vi "ArrayFunctions_CheckForDups(DBL).vi"(1 "Array":dbl[](array[numeric])) -> (15 "DupElements":dbl[](array[numeric]), 16 "DupElements(String)":string, 17 "FoundDups":bool)   [LabVIEW 2016]
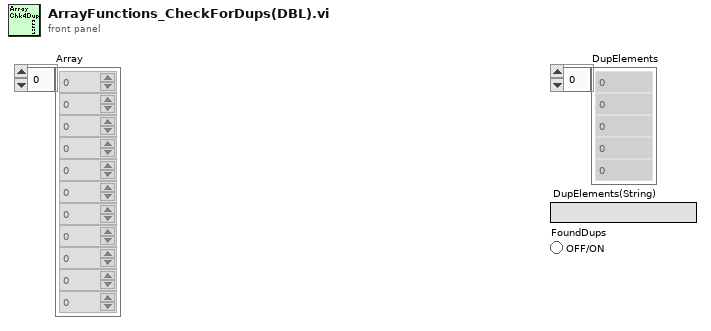
[diagram p1: front panel]
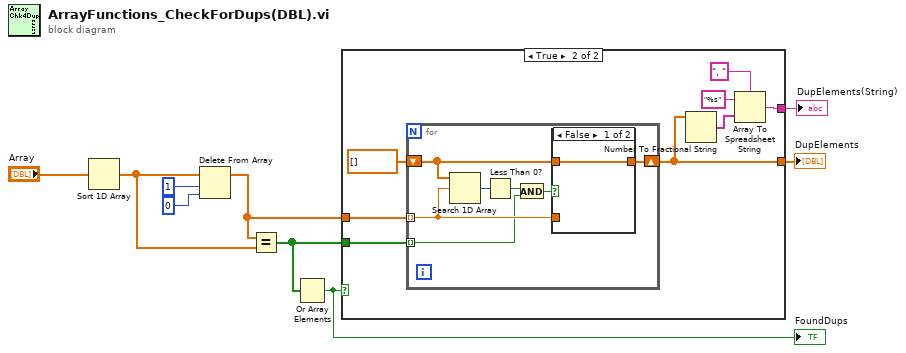
[diagram p0: block diagram]
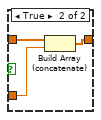
[diagram p3: hidden frame]
diagram:
  n1 = Sort 1D Array(array="Array") -> (sorted array=w2:dbl[])
  n2 = Delete From Array(array=w2, length=1, index=0) -> (array with subset deleted=w7:dbl[])  [unwired: 1 out]
  n3 = Equal?(x=w7, y=w2) -> (x = y?=w6:bool[])
  n4 = Or Array Elements(Boolean array=w6) -> (logical OR=w4:bool)
  "FoundDups" <- w4
  n5 = case shown="True" w4 {
    tunnel: w7 -> [_ w17]
    tunnel: w6 -> [_ w16]
    tunnel: [_ w14] -> w5
    tunnel: [_ w10] -> w1
    frame False {
    }
    frame True {
      n6 = for {
        tunnel: w17 -> [w22] mode=indexing
        tunnel: w16 -> [w18] mode=indexing
        shift-right: [w24] -> w14
        shift-left: dbl[] [] ("array w/ subset deleted") -> [w23]
        n7 = Search 1D Array(1D array=w23, element=w22) -> (index of element=w21:i32)  [unwired: 1 in]
        n8 = Less Than 0?(x=w21) -> (x < 0?=w20:bool)
        n9 = And(x=w20, y=w18) -> (x .and. y?=w19:bool)
        n10 = case shown="False" w19 {
          tunnel: [w25 w28] -> w24
          tunnel: w23 -> [w25 w27]
          tunnel: w22 -> [_ w26]
          frame False {
          }
          frame True {
            n11 = Build Array (concatenate)(w27, w26) -> (w28:dbl[])
          }
        }
      }
      n12 = Number To Fractional String(number=w14) -> (F-format string=w11:string[])  [unwired: 3 in]
      n13 = Array To Spreadsheet String(delimiter (Tab)=", ", array=w11, 3:"%s" ("format string")) -> (spreadsheet string=w10:string)
    }
  }
  "DupElements" <- w5
  "DupElements(String)" <- w1
